vi "GUILib.VI-Tree.vi"() -> ()   [LabVIEW 2012, in "GUILib.lvlib"]
doc: "Contains VIs intended for programming. \n\nauthor and license: GPL, see description of owning library."
uses:
  GUILib.lvlib
  GUILib.simpleBoolean.ctl
  GUILib.basicBoolean.ctl
  GUILib.simpleNumeric.ctl
  GUILib.basicNumeric.ctl
  GUILib.userEventsMainType.ctl
panel:
  in  "userEventsMain":T1
  in  "simpleNumeric":T2 {"nom" step=22.0}
  in  "simpleBoolean":T4
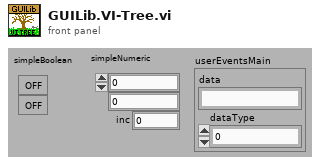
[diagram p1: front panel]
types:
  T1 = typedef "GUILib.lvlib/GUILib.userEventsMainType.ctl" = cluster{"data":string, "dataType":i32}
  T2 = typedef "GUILib.lvlib/GUILib.simpleNumeric.ctl" = cluster{"nom":T3, "act":dbl, "inc":dbl}
  T3 = typedef "GUILib.lvlib/GUILib.basicNumeric.ctl" = dbl
  T4 = typedef "GUILib.lvlib/GUILib.simpleBoolean.ctl" = cluster{"nominal":T5, "actual":T5}
  T5 = typedef "GUILib.lvlib/GUILib.basicBoolean.ctl" = bool
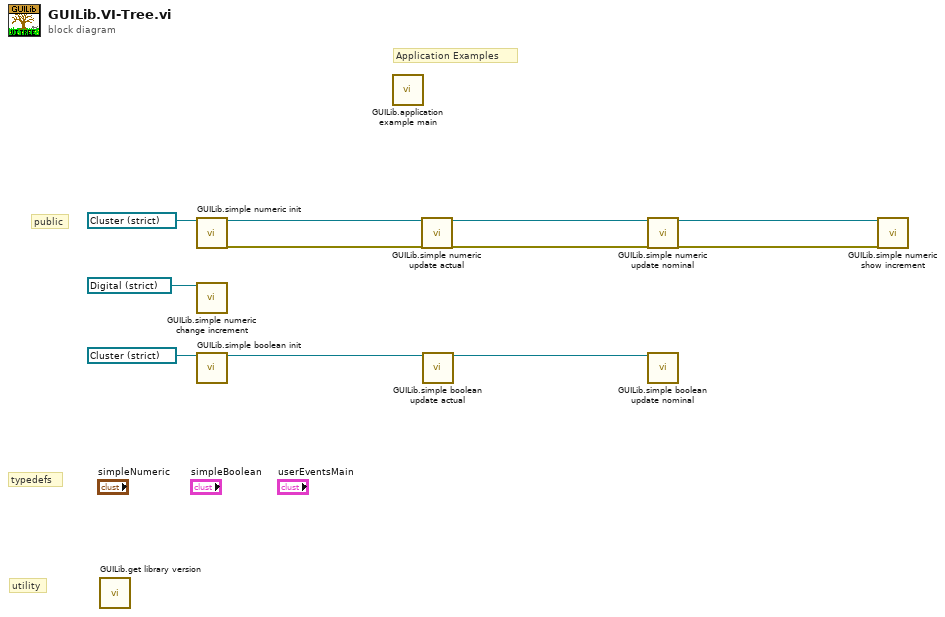
[diagram p0: block diagram]
diagram:
  # "utility"
  # "typedefs"
  # "Application Examples"
  # "public"
  n1 = call "GUILib.get library version.vi"() -> ()  [unwired: 1 in, 1 out]
  n2 = call "GUILib.simple numeric init.vi"("ctlRef"=refnum<vi> refnum) -> ("ctlRef dup"=w9:refnum<vi>, "error out"=w7:errorcluster)  [unwired: 17 in]
  n3 = call "GUILib.simple numeric change increment.vi"("ctlRef"=refnum<vi> refnum) -> ()  [unwired: 17 in, 2 out]
  n4 = call "GUILib.simple boolean init.vi"("ctlRef"=refnum<vi> refnum) -> ("ctlRef dup"=w3:refnum<vi>)  [unwired: 17 in, 1 out]
  n5 = call "GUILib.application example main.vi"() -> ()  [unwired: 1 in]
  n6 = call "GUILib.simple numeric update actual.vi"("ctlRef"=w9, "error in (no error)"=w7) -> ("ctlRef out"=w8:refnum<vi>, "error out"=w6:errorcluster)  [unwired: 16 in]
  n7 = call "GUILib.simple boolean update actual.vi"("ctlRef"=w3) -> ("ctlRef out"=w4:refnum<vi>)  [unwired: 17 in, 1 out]
  n8 = call "GUILib.simple numeric update nominal.vi"("ctlRef"=w8, "error in (no error)"=w6) -> ("ctlRef out"=w2:refnum<vi>, "error out"=w1:errorcluster)  [unwired: 16 in]
  n9 = call "GUILib.simple boolean update nominal.vi"("ctlRef"=w4) -> ()  [unwired: 17 in, 2 out]
  n10 = call "GUILib.simple numeric show increment.vi"("ctlRef"=w2, "error in (no error)"=w1) -> ()  [unwired: 16 in, 2 out]
